vi "NXT Stay Awake.vi"(2 "error in (no error)":errorcluster, 3 "Sys Call Refnum":T1) -> (0 "error out":errorcluster)   [LabVIEW 2012, in "ENGR3390 Tug Boat.lvrbt"]
doc: "This VI resets the NXT Keep Alive timer to zero to prevent the NXT from shutting down when running without a front button push."
uses:
  <vilib>/NXT/NXT Controls/NXTSyscallRefnum.ctl
  ENGR3390 Tug Boat.lvrbt
  <resource>/objmgr/NXTInputOutput.rc
panel:
  out "NXTKeepAlive":u32
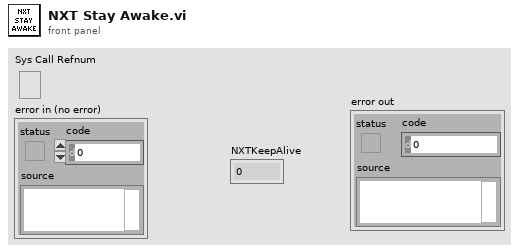
[diagram p1: front panel]
types:
  T1 = typedef "NXTSyscallRefnum.ctl" = refnum<k21>
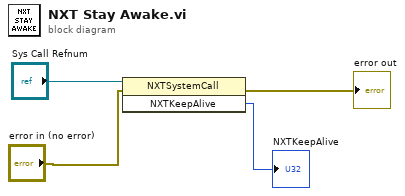
[diagram p0: block diagram]
diagram:
  n1 = invoke class="NXTSystemCall" method="NXTKeepAlive"(reference="Sys Call Refnum", error in="error in (no error)") -> (error out=→"error out":errorcluster, "NXTKeepAlive"=→"NXTKeepAlive":u32)  [unwired: 1 in, 1 out]
